vi "test item and extname.vi"(10 "tpdata":string[](array[string])) -> (2 "Nxt.Name":string[](array[string]), 3 "test item":string[](array[string]))   [LabVIEW 2018]
panel:
  out "数组":string[](array[string])
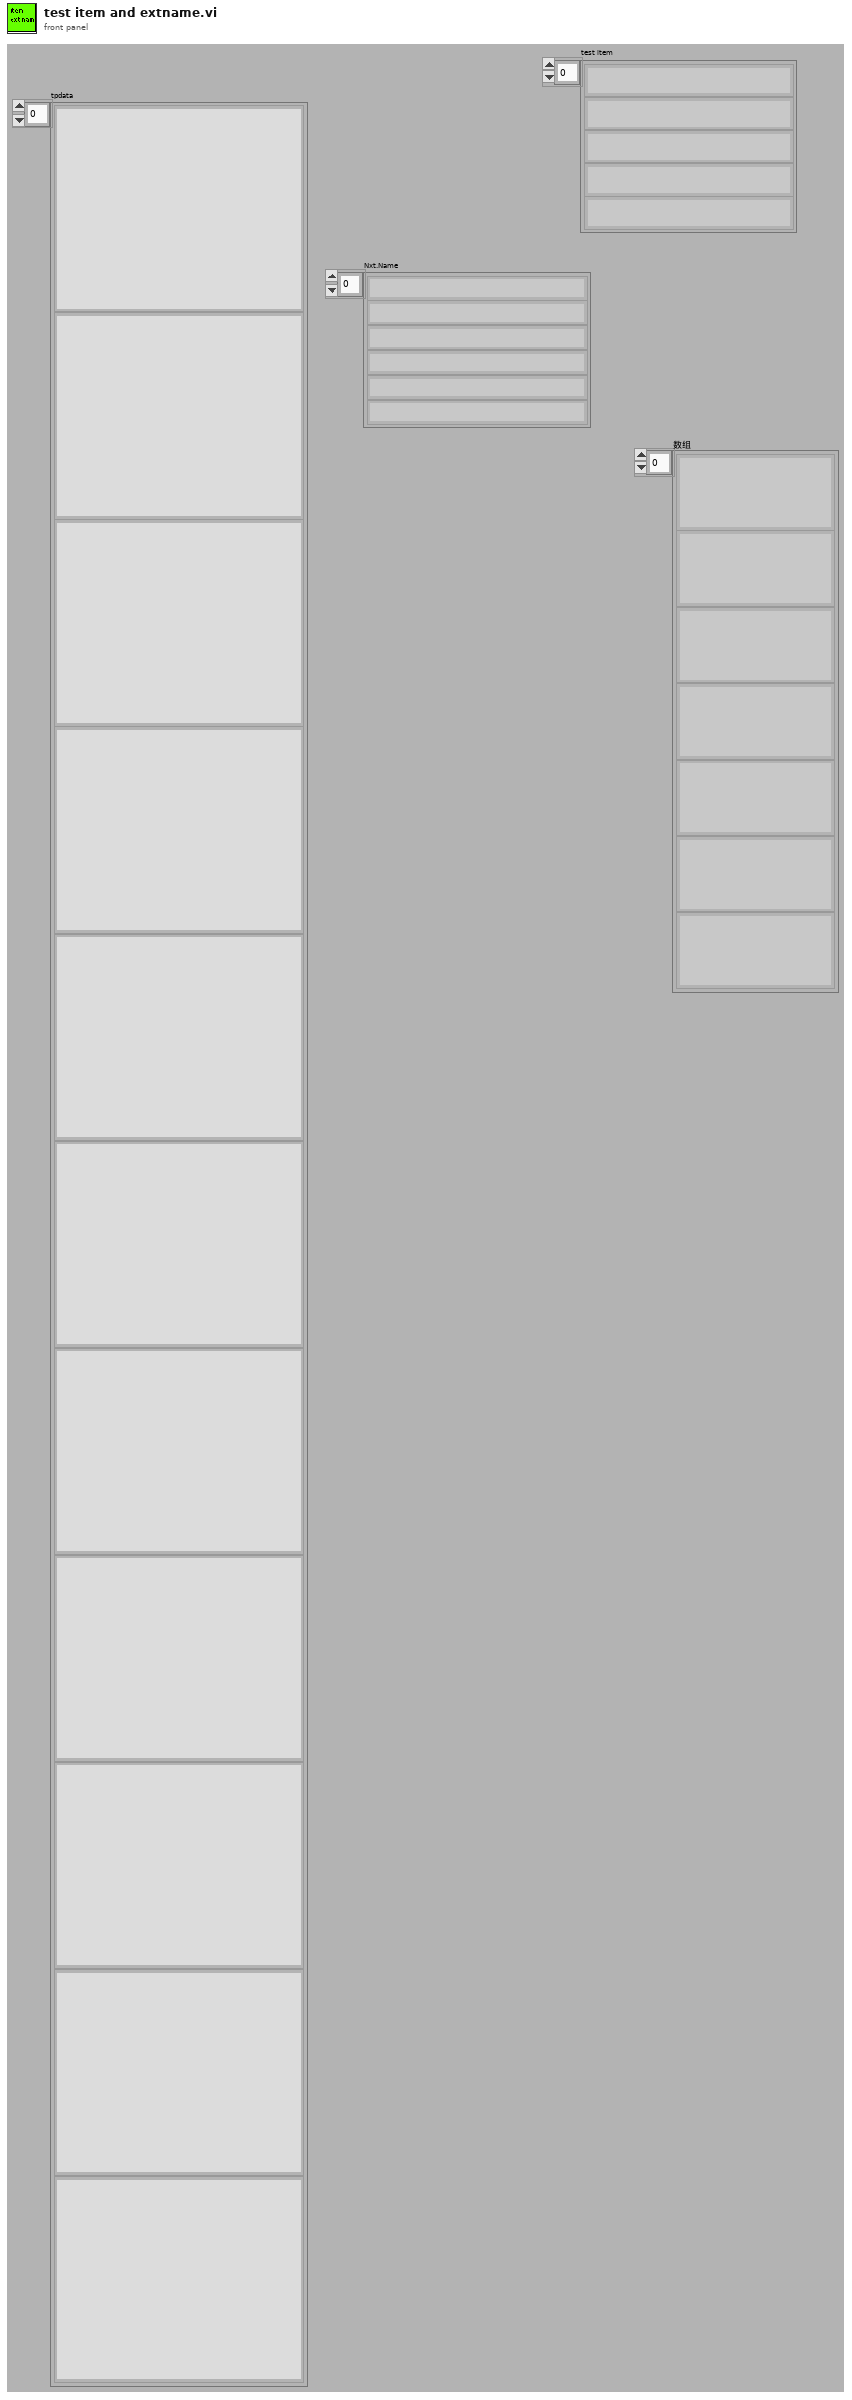
[diagram p1: front panel]
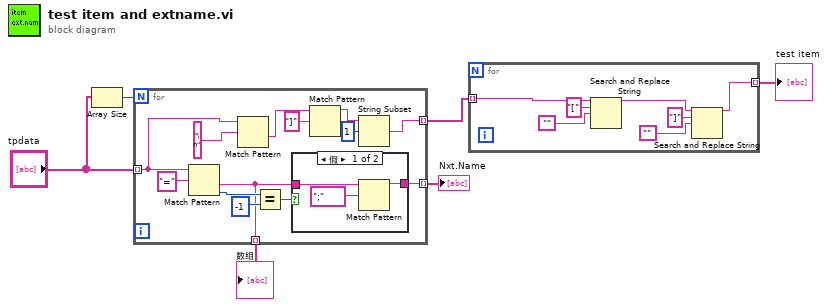
[diagram p0: block diagram]
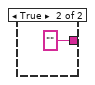
[diagram p2: hidden frame]
diagram:
  n1 = Array Size(array="tpdata") -> (size(s)=w6:i32)
  n2 = for {
    N: w6 -> [_]
    tunnel: "tpdata" -> [w9] mode=indexing
    tunnel: [w15] -> w5 mode=indexing
    tunnel: [w8] -> w2 mode=indexing
    tunnel: [w10] -> w4 mode=indexing
    n3 = Match Pattern(string=w9, regular expression="=") -> (after substring=w10:string, offset past match=w18:i32)  [unwired: 3 out]
    n4 = Match Pattern(string=w9, regular expression="\n") -> (after substring=w14:string)  [unwired: 4 out]
    n5 = Equal?(x=w18, y=-1) -> (x = y?=w16:bool)
    n6 = case shown="假" w16 {
      tunnel: [w20 ""] -> w15
      tunnel: w10 -> [w22 _]
      frame False {
        n7 = Match Pattern(string=w22, regular expression=";") -> (before substring=w20:string)  [unwired: 4 out]
      }
      frame True {
      }
    }
    n8 = Match Pattern(string=w14, regular expression="]" ("正则表达式")) -> (before substring=w12:string)  [unwired: 4 out]
    n9 = String Subset(string=w12, offset (0)=1 ("偏移量(0)")) -> (substring=w8:string)  [unwired: 1 out]
  }
  "Nxt.Name" <- w5
  "数组" <- w4
  n10 = for {
    tunnel: w2 -> [w30] mode=indexing
    tunnel: [w24] -> w1 mode=indexing
    n11 = Search and Replace String(input string=w30, search string="[" ("搜索字符串"), replace string="") -> (result string=w25:string)  [unwired: 5 in, 3 out]
    n12 = Search and Replace String(input string=w25, search string="]" ("搜索字符串"), replace string="") -> (result string=w24:string)  [unwired: 5 in, 3 out]
  }
  "test item" <- w1
